vi "Get Slave IOVs.vi"(8 "error in (no error)":errorcluster, 11 "ECAT Master in":refnum<k21>) -> (0 "error IO":errorcluster, 2 "All Slaves":refnum<k21>[](array[refnum]), 3 "ECAT Master out":refnum<k21>)   [LabVIEW 2020, in "SEECD Engine.lvlib"]
uses:
  SEECD Engine.lvlib
  <resource>/objmgr/IndComECAT.rc
  Shared/SEECD Shared.lvlib
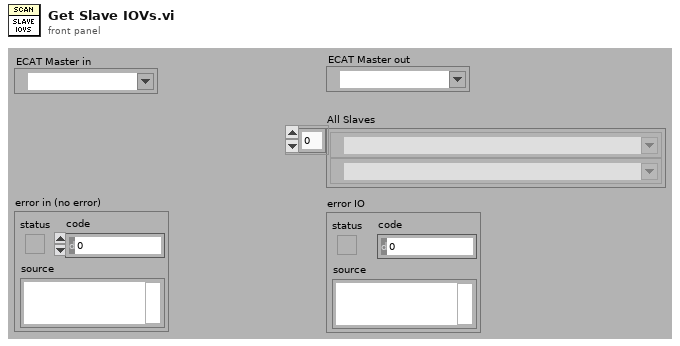
[diagram p1: front panel]
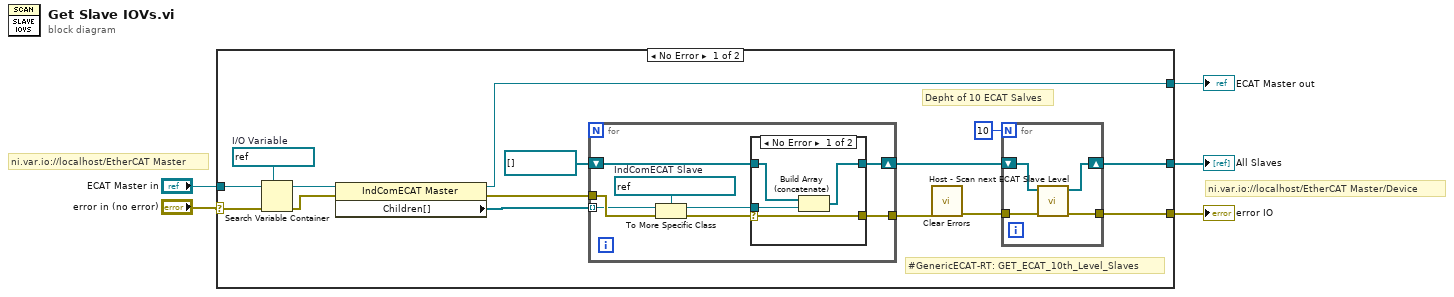
[diagram p0: block diagram]
diagram:
  # "ni.var.io://localhost/EtherCAT Master/Device"
  # "ni.var.io://localhost/EtherCAT Master"
  n1 = case shown="No Error" "error in (no error)" {
    selector: "error in (no error)" -> [w12 w40]
    tunnel: [w6 w40] -> w5
    tunnel: "ECAT Master in" -> [w13 w39]
    tunnel: [w20 w39] -> w3
    tunnel: [w9 _] -> w1
    frame No Error {
      w14 = refnum<k21> refnum  # I/O Variable
      # "#GenericECAT-RT: GET_ECAT_10th_Level_Slaves"
      # "Depht of 10 ECAT Salves"
      n2 = Search Variable Container(7:w14, 8:w12, 11:w13) -> (0:w11:errorcluster, 3:w10:refnum<k21>)  [unwired: 3 in, 1 out]
      n3 = property class="IndComECAT Master"(reference=w10, error in=w11) -> (reference out=w20:refnum<k21>, error out=w8:errorcluster, "Children[]"=w7:refnum<k21>[])
      n4 = for {
        tunnel: w7 -> [w27] mode=indexing
        tunnel: w8 -> [w28]
        shift-right: [w25] -> w15
        shift-left: refnum<k21>[] [] -> [w24]
        tunnel: [w23] -> w18
        w26 = refnum<k21> refnum  # IndComECAT Slave
        n5 = To More Specific Class(target class=w26, reference=w27, error in=w28) -> (specific class reference=w21:refnum<k21>, error out=w22:errorcluster)
        n6 = case shown="No Error" w22 {
          selector: w22 -> [w30 w33]
          tunnel: w21 -> [w29 _]
          tunnel: [w32 w34] -> w25
          tunnel: w24 -> [w31 w34]
          tunnel: [w30 w33] -> w23
          frame No Error {
            n7 = Build Array (concatenate)(w31, w29) -> (w32:refnum<k21>[])
          }
          frame Error {
          }
        }
      }
      n8 = call <vilib>:"Clear Errors.vi"("error in (no error)"=w18) -> ("error out"=w16:errorcluster)  [unwired: 5 in, 1 out]
      n9 = for {
        N: 10 -> [_]
        tunnel: w16 -> [w38]
        tunnel: [w36] -> w6
        shift-right: [w37] -> w9
        shift-left: w15 -> [w35]
        n10 = call "Host - Scan next ECAT Slave Level.vi"("Fehler (Eingang, kein Fehler)"=w38, "Array (Eingang)"=w35) -> ("Fehler (Ausgang)"=w36:errorcluster, "Array (Ausgang)"=w37:refnum<k21>[])  [unwired: 8 in]
      }
    }
    frame Error {
    }
  }
  "All Slaves" <- w1
  "error IO" <- w5
  "ECAT Master out" <- w3
